vi "Read New Camera Parameters.vi"(8 "error in (no error)":errorcluster, 11 "Image Undistorter in":refnum<class "Image Undistorter.lvclass">) -> (0 "error out":errorcluster, 2 "Camera Parameters":T1, 3 "Image Undistorter":refnum<class "Image Undistorter.lvclass">)   [LabVIEW 2020, in "image.lvlib" / "Image Undistorter.lvclass"]
doc: "Get the Camera Matrix for the Camera that would provide the undistorted image."
uses:
  Image Undistorter.lvclass
  Image Undistorter.lvclass/Image Undistorter.ctl
  common/Camera Matrix.ctl
  common/common.lvlib
  common/Camera Distortion Coefficients.ctl
  common/Camera Parameters.ctl
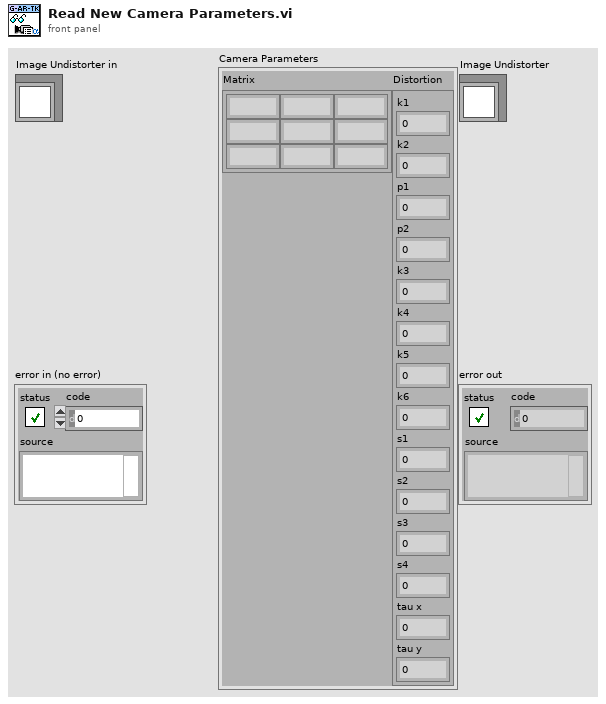
[diagram p1: front panel]
types:
  T1 = typedef "common.lvlib/Camera Parameters.ctl" = cluster{"Matrix":T2, "Distortion":T3}
  T2 = typedef "common.lvlib/Camera Matrix.ctl" = cluster{"m 0,0":dbl, "m 0,1":dbl, "m 0,2":dbl, "m 1,0":dbl, "m 1,1":dbl, "m 1,2":dbl, "m 2,0":dbl, "m 2,1":dbl, "m 2,2":dbl}
  T3 = typedef "common.lvlib/Camera Distortion Coefficients.ctl" = cluster{"k1":dbl, "k2":dbl, "p1":dbl, "p2":dbl, "k3":dbl, "k4":dbl, "k5":dbl, "k6":dbl, "s1":dbl, "s2":dbl, "s3":dbl, "s4":dbl, "tau x":dbl, "tau y":dbl}
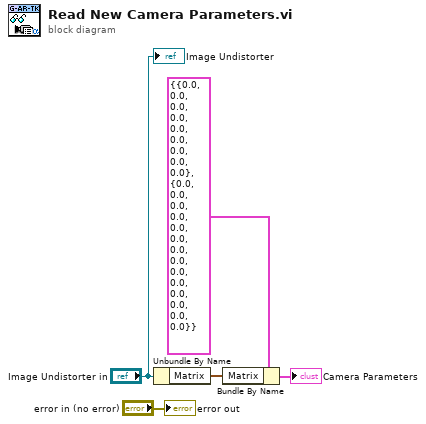
[diagram p0: block diagram]
diagram:
  n1 = Unbundle By Name("Image Undistorter in") -> ("Matrix"=w2:T2)
  n2 = Bundle By Name(cluster=T1 {"Matrix"={"m 0,0"=0.0, "m 0,1"=0.0, "m 0,2"=0.0, "m 1,0"=0.0, "m 1,1"=0.0, "m 1,2"=0.0, "m 2,0"=0.0, "m 2,1"=0.0, "m 2,2"=0.0}, "Distortion"={"k1"=0.0, "k2"=0.0, "p1"=0.0, "p2"=0.0, "k3"=0.0, "k4"=0.0, "k5"=0.0, "k6"=0.0, "s1"=0.0, "s2"=0.0, "s3"=0.0, "s4"=0.0, "tau x"=0.0, "tau y"=0.0}} ("Camera Parameters"), "Matrix"=w2) -> (→"Camera Parameters":T1)
  "error out" <- "error in (no error)"
  "Image Undistorter" <- "Image Undistorter in"
